vi "Close Wfm Sessions.vi"(8 "Error In":errorcluster, 11 "Async State Vars":T1) -> (0 "Error Out":errorcluster)   [LabVIEW 2017, in "Waveform-Processing-Custom-Device Engine.lvlib"]
uses:
  Waveform-Processing-Custom-Device Engine.lvlib
  Types/AsyncStateVariables.ctl
  <vilib>/NI Veristand/Custom Device Waveform API/Single Waveform Read (DBL)/Single Waveform Read (DBL).lvclass
  <vilib>/NI Veristand/Custom Device Waveform API/Single Waveform Write (DBL)/Single Waveform Write (DBL).lvclass
  <vilib>/NI Veristand/Custom Device API/Waveform Data Reference.ctl
  Types/New Async FIFOs.ctl
  <vilib>/NI/NIVS Inline Async API/_Data Access Engine/Data Access Engine/Types/Write.DVR.ctl
  <vilib>/NI/NIVS Inline Async API/_Data Access Engine/Access Type Classes/Write/Write.lvclass
  <vilib>/NI/NIVS Inline Async API/_Data Access Engine/Data Access Engine/Types/Read.DVR.ctl
  <vilib>/NI/NIVS Inline Async API/_Data Access Engine/Access Type Classes/Read/Read.lvclass
  <vilib>/NI Veristand/Custom Device Waveform API/Single Waveform Read (DBL)/NI VeriStand - Close Single Waveform Read Session (DBL).vi
  <vilib>/NI Veristand/Custom Device Waveform API/Single Waveform Write (DBL)/NI VeriStand - Close Single Waveform Write Session (DBL).vi
  <vilib>/NI Veristand/Custom Device Waveform API/NI_VS Custom Device Waveform API.lvlib
  <vilib>/NI Veristand/Custom Device API/Custom Device API.lvlib
  <vilib>/NI/NIVS Inline Async API/_Data Access Engine/Data Access Engine/Data Access Engine.lvclass
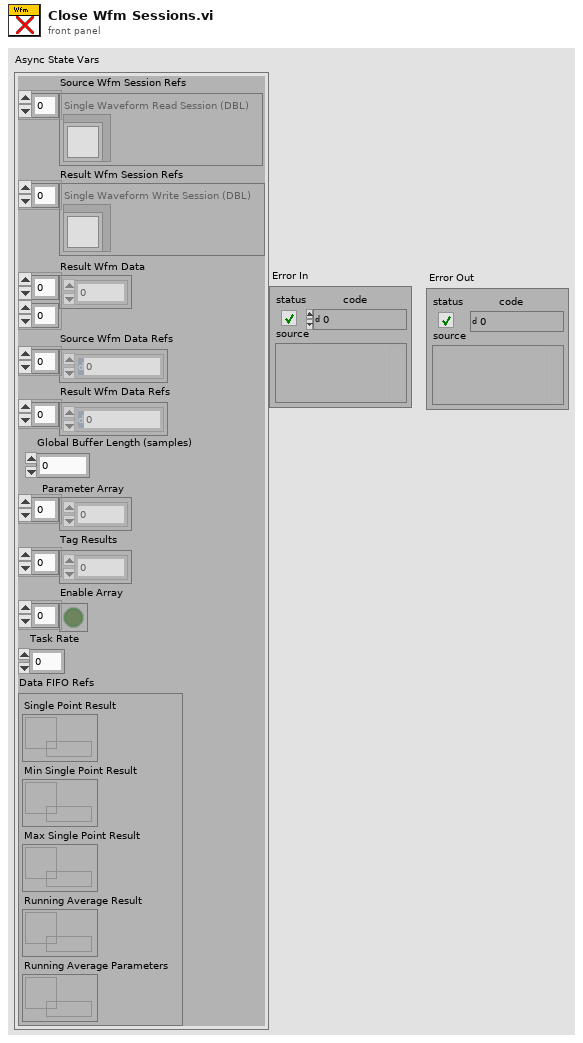
[diagram p1: front panel]
types:
  T1 = typedef "Waveform-Processing-Custom-Device Engine.lvlib/AsyncStateVariables.ctl" = cluster{"Source Wfm Session Refs":refnum<class "Single Waveform Read (DBL).lvclass">[], "Result Wfm Session Refs":refnum<class "Single Waveform Write (DBL).lvclass">[], "Result Wfm Data":dbl[][], "Source Wfm Data Refs":T2[], "Result Wfm Data Refs":T2[], "Global Buffer Length (samples)":dbl, "Parameter Array":dbl[], "Tag Results":dbl[], "Enable Array":bool[], "Task Rate":dbl, "Data FIFO Refs":T3}
  T2 = typedef "Custom Device API.lvlib/Waveform Data Reference.ctl" = i32
  T3 = typedef "Waveform-Processing-Custom-Device Engine.lvlib/New Async FIFOs.ctl" = cluster{"Single Point Result":T4, "Running Average Result":T4, "Running Average Parameters":T5, "Min Single Point Result":T4, "Max Single Point Result ":T4}
  T4 = typedef "Data Access Engine.lvlib/Data Access Engine.lvclass/Write.DVR.ctl" = refnum<data-value>
  T5 = typedef "Data Access Engine.lvlib/Data Access Engine.lvclass/Read.DVR.ctl" = refnum<data-value>
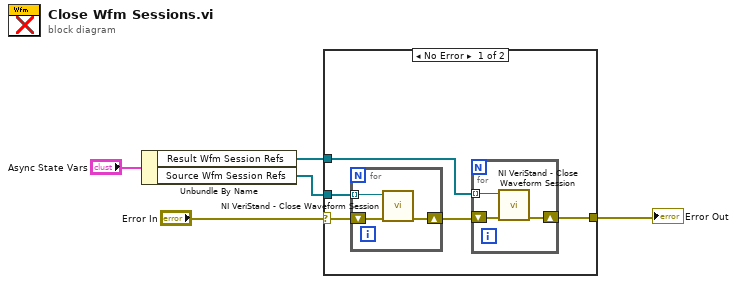
[diagram p0: block diagram]
diagram:
  n1 = Unbundle By Name("Async State Vars") -> ("Result Wfm Session Refs"=w2:refnum<class "Single Waveform Write (DBL).lvclass">[], "Source Wfm Session Refs"=w1:refnum<class "Single Waveform Read (DBL).lvclass">[])
  n2 = case shown="No Error" "Error In" {
    selector: "Error In" -> [w10 w17]
    tunnel: [w8 w17] -> w4
    tunnel: w2 -> [w6 _]
    tunnel: w1 -> [w7 _]
    frame No Error {
      n3 = for {
        tunnel: w7 -> [w14] mode=indexing
        shift-right: [w15] -> w9
        shift-left: w10 -> [w16]
        n4 = call-poly <vilib>:"NI VeriStand - Close Waveform Session.vi"("error in (no error)"=w16, "Single Waveform Read Session (DBL)"=w14) -> ("error out"=w15:errorcluster)  [unwired: 9 in]
      }
      n5 = for {
        tunnel: w6 -> [w11] mode=indexing
        shift-right: [w12] -> w8
        shift-left: w9 -> [w13]
        n6 = call-poly <vilib>:"NI VeriStand - Close Waveform Session.vi"("error in (no error)"=w13, "Single Waveform Write Session (DBL)"=w11) -> ("error out"=w12:errorcluster)  [unwired: 9 in]
      }
    }
    frame Error {
    }
  }
  "Error Out" <- w4
